vi "BELKIN Read Dest FIFO.vi"(7 "Read Timeout (ms)":i32=5000, 8 "error in (no error)":errorcluster, 9 "FPGA VI Reference In":refnum<k20>, 10 "Maximum Pixels per Read":i32=-1, 11 "Image":T1) -> (0 "error out":errorcluster, 1 "FPGA VI Reference Out":refnum<k20>, 3 "Image Out":T1)   [LabVIEW 2015]
doc: "Transfers an image from the target FPGA to the host processor via DMA FIFO."
uses:
  <vilib>/vision/Image Controls.llb/IMAQ Image.ctl
  <vilib>/rvi/errors/niLvFpgaAdjustHostInterfaceError.vi
  <vilib>/rvi/interface/nirviMethod/nirviMethod.xnode
  <vilib>/rvi/errors/niLvFpgaMergeErrorWithErrorCode.vi
  <vilib>/vision/EDVR.llb/IMAQ ImageToEDVR 2D U8.vi
  nivissvc.dll
  <vilib>/FPGAPlugInAG/Dynamic/niLvFpga_ReadFifo_Dynamic.vi
  <vilib>/FPGAPlugInAG/Dynamic/niLvFpga_AcquireReadRegionFifo_Dynamic.vi
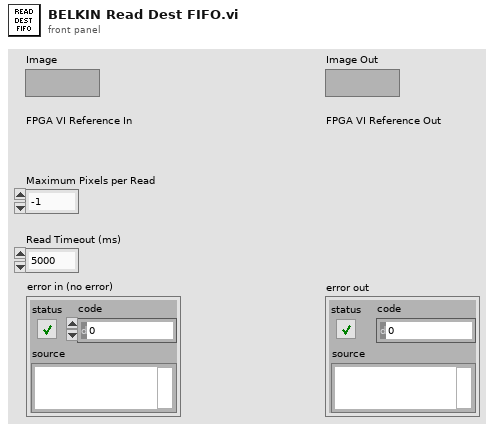
[diagram p1: front panel]
types:
  T1 = typedef "IMAQ Image.ctl" = refnum<image>
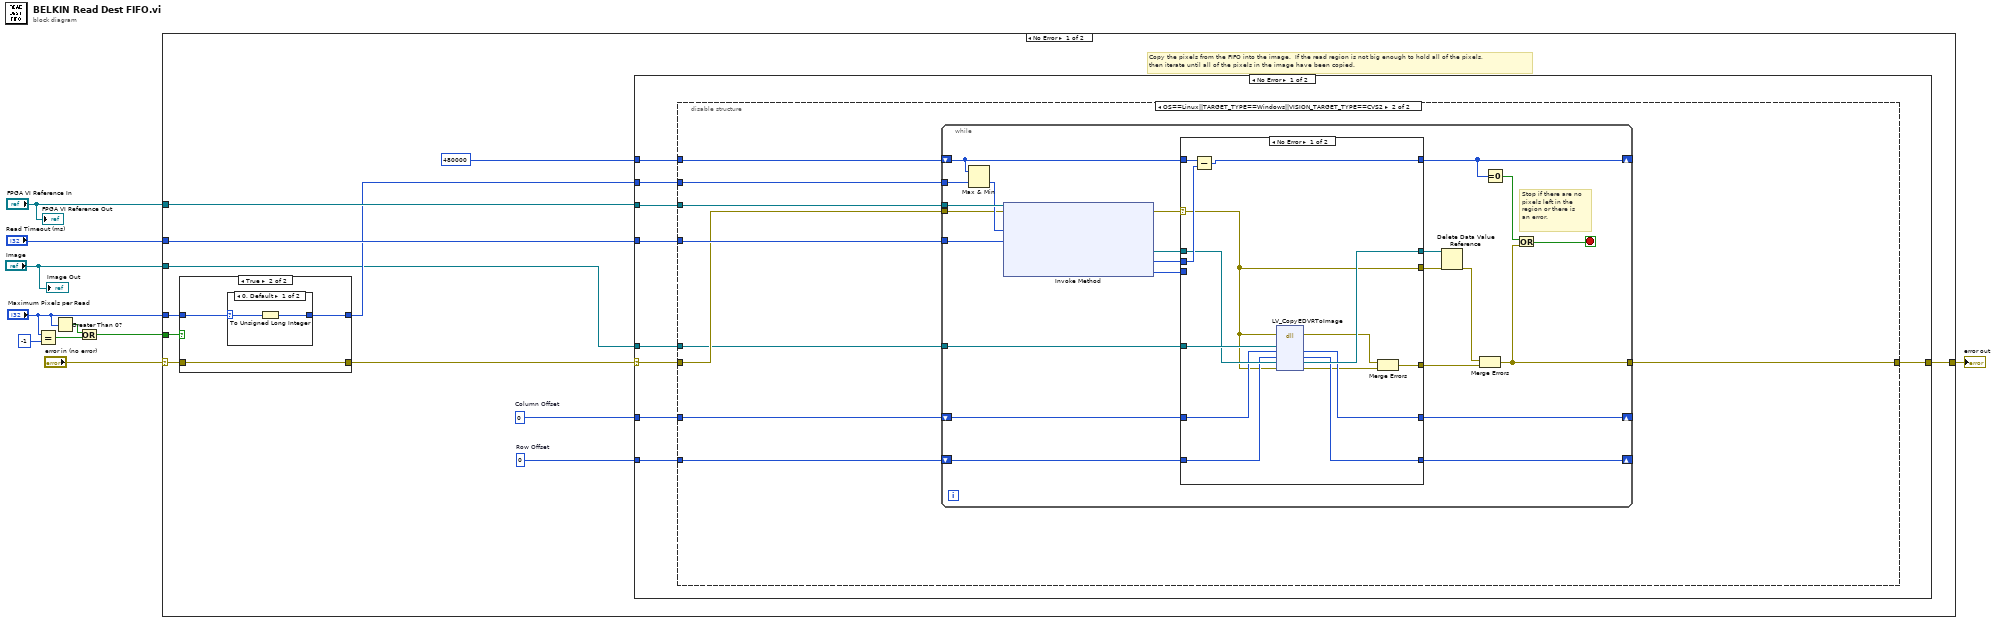
[diagram p0: block diagram]
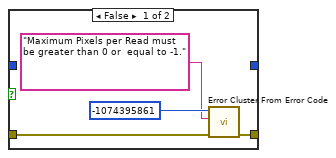
[diagram p2: hidden frame]
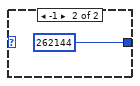
[diagram p3: hidden frame]
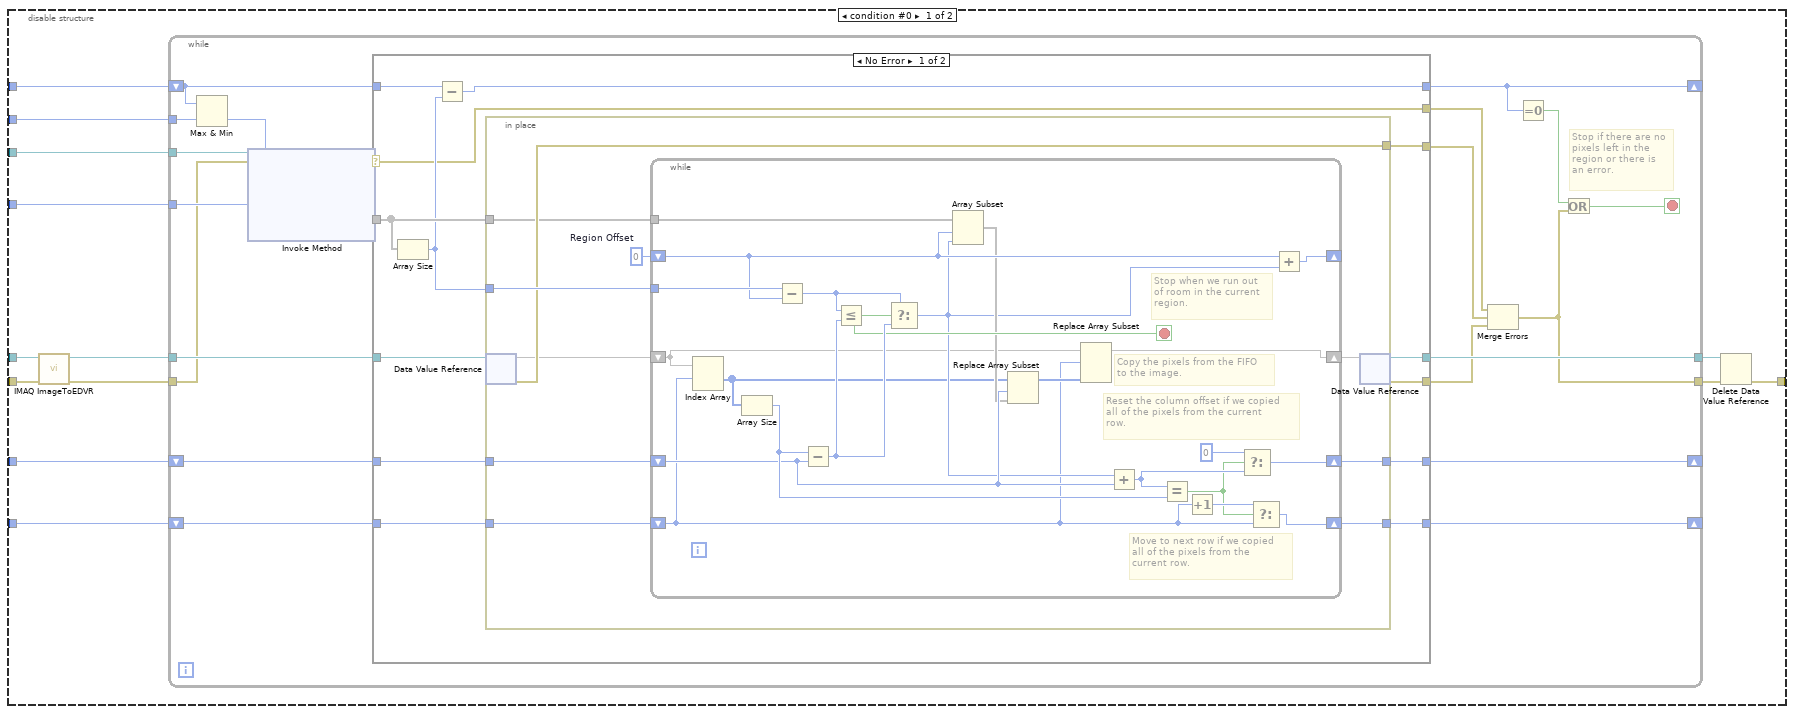
[diagram p4: hidden frame]
diagram:
  n1 = Equal?(x="Maximum Pixels per Read", y=-1) -> (x = y?=w6:bool)
  n2 = Greater Than 0?(x="Maximum Pixels per Read") -> (x > 0?=w7:bool)
  n3 = Or(x=w7, y=w6) -> (x .or. y?=w5:bool)
  n4 = case shown="No Error" "error in (no error)" {
    selector: "error in (no error)" -> [w12 w178]
    tunnel: "FPGA VI Reference In" -> [w20 _]
    tunnel: "Read Timeout (ms)" -> [w19 _]
    tunnel: w5 -> [w18 _]
    tunnel: "Maximum Pixels per Read" -> [w17 _]
    tunnel: "Image" -> [w14 _]
    tunnel: [w13 w178] -> w2
    frame No Error {
      w21 = u32 0  # Row Offset
      w22 = u32 0  # Column Offset
      # "Copy the pixels from the FIFO into the image.  If the read region is not big enough to hold all of the pixels,\nthen iterate until all of the pixels in the image have been copied."
      n5 = case shown="True" w18 {
        tunnel: w12 -> [w24 w29]
        tunnel: [w23 w29] -> w16
        tunnel: w17 -> [_ w28]
        tunnel: [_ w27] -> w15
        frame False {
          n6 = call <vilib>:"Error Cluster From Error Code.vi"("error in (no error)"=w24, "error message (\"\")"="Maximum Pixels per Read must be greater than 0 or  equal to -1." ("error message (\"\")"), "error code (0)"=-1074395861) -> ("error out"=w23:errorcluster)  [unwired: 6 in]
        }
        frame True {
          n7 = case shown="0, Default" w28 {
            selector: w28 -> [w31 _]
            tunnel: [w30 u32 262144 ("Maximum Pixels per Write")] -> w27
            frame 0, Default {
              n8 = To Unsigned Long Integer(number=w31) -> (unsigned 32bit integer=w30:u32)
            }
            frame -1 {
            }
          }
        }
      }
      n9 = case shown="No Error" w16 {
        selector: w16 -> [w40 w177]
        tunnel: 480000 ("x*y") -> [w34 _]
        tunnel: w22 -> [w39 _]
        tunnel: w21 -> [w38 _]
        tunnel: w20 -> [w36 _]
        tunnel: [w33 w177] -> w13
        tunnel: w15 -> [w35 _]
        tunnel: w19 -> [w37 _]
        tunnel: w14 -> [w41 _]
        frame No Error {
          n10 = disable-structure shown="OS==Linux||TARGET_TYPE==Windows||VISION_TARGET_TYPE==CVS2" {
            disable-tunnel: w34 -> [w54 w134]
            disable-tunnel: w39 -> [w53 w133]
            disable-tunnel: w38 -> [w52 w132]
            disable-tunnel: w36 -> [w51 w131]
            disable-tunnel: [w42 w130] -> w33
            disable-tunnel: w35 -> [w50 w129]
            disable-tunnel: w37 -> [w49 w128]
            disable-tunnel: w41 -> [w48 w126]
            disable-tunnel: w40 -> [w46 w127]
            frame condition #0 {
              n11 = call-poly <vilib>:"IMAQ ImageToEDVR.vi"("error in (no error)"=w46, "Image"=w48) -> ("error out"=w45:errorcluster, "EDVR 2D U8"=w47:refnum<data-value>)  [unwired: 7 in, 1 out]
              n12 = while {
                shift-right: [w66] -> _
                shift-left: w54 -> [w62]
                shift-right: [w71] -> _
                shift-left: w53 -> [w73]
                shift-right: [w74] -> _
                shift-left: w52 -> [w72]
                tunnel: w51 -> [w70]
                tunnel: [w68] -> w44
                tunnel: [w64] -> w43
                tunnel: w50 -> [w60]
                tunnel: w49 -> [w59]
                tunnel: w47 -> [w56]
                tunnel: w45 -> [w55]
                stop <- w65 stop-if-true
                # "Stop if there are no\npixels left in the \nregion or there is\nan error."
                n13 = Max & Min(x=w62, y=w60) -> (min(x,y)=w61:u32)  [unwired: 1 out]
                n14 = xnode "Invoke Method"("FPGA VI Reference In"=w70, "error in"=w55, "Number of Elements"=w61, "Timeout (ms)"=w59) -> ("error out"=w69:errorcluster, "Data"=w75:void[])  [unwired: 2 out]
                n15 = case shown="No Error" w69 {
                  selector: w69 -> [w76 w121]
                  tunnel: w62 -> [w88 w124]
                  tunnel: [w87 w124] -> w66
                  tunnel: w56 -> [w86 w125]
                  tunnel: w75 -> [w78 _]
                  tunnel: [w85 w122] -> w74
                  tunnel: w73 -> [w84 w123]
                  tunnel: w72 -> [w83 w122]
                  tunnel: [w82 w123] -> w71
                  tunnel: [w81 w125] -> w68
                  tunnel: [w76 w121] -> w58
                  tunnel: [w80 _] -> w57
                  tunnel: [w79 _] -> w67
                  frame No Error {
                    n16 = Array Size(array=w78) -> (size(s)=w77:i32)
                    n17 = Subtract(x=w88, y=w77) -> (x-y=w87:i32)
                    n18 = in-place {
                      in-place-border: w77 -> [w96]
                      in-place-border: [w98] -> w85
                      in-place-border: w84 -> [w95]
                      in-place-border: w83 -> [w91]
                      in-place-border: [w94] -> w82
                      in-place-border: [w93] -> w79
                      in-place-border: w78 -> [w89]
                      w97 = u32 0  # Region Offset
                      n19 = in-place-dvr #1(w86) -> (w92:u8[][], w93:errorcluster)
                      n20 = while {
                        shift-right: [w118] -> _
                        shift-left: w97 -> [w117]
                        tunnel: w89 -> [w107]
                        tunnel: w96 -> [w120]
                        shift-right: [w112] -> w94
                        shift-left: w95 -> [w108]
                        shift-right: [w99] -> w90
                        shift-left: w92 -> [w102]
                        shift-right: [w110] -> w98
                        shift-left: w91 -> [w100]
                        stop <- w109 stop-if-true
                        # "Stop when we run out\nof room in the current\nregion."
                        # "Copy the pixels from the FIFO\nto the image."
                        # "Reset the column offset if we copied\nall of the pixels from the current\nrow."
                        # "Move to next row if we copied\nall of the pixels from the\ncurrent row."
                        n21 = Index Array(array=w102, index (row)=w100) -> (element=w103:u8[])  [unwired: 1 in]
                        n22 = Array Size(array=w103) -> (size(s)=w116:i32)
                        n23 = Subtract(x=w120, y=w117) -> (x-y=w119:u32)
                        n24 = Subtract(x=w116, y=w108) -> (x-y=w115:u32)
                        n25 = Less Or Equal?(x=w119, y=w115) -> (x <= y?=w109:bool)
                        n26 = Select(t=w119, s=w109, f=w115) -> (s? t:f=w105:u32)
                        n27 = Array Subset(array=w107, index=w117, length=w105) -> (w106:void[])
                        n28 = Replace Array Subset(array=w103, new element=w106, index=w108) -> (w101:u8[])
                        n29 = Replace Array Subset(array=w102, new element=w101, index (row)=w100) -> (w99:u8[][])  [unwired: 1 in]
                        n30 = Add(x=w105, y=w108) -> (x+y=w113:u32)
                        n31 = Equal?(x=w113, y=w116) -> (x = y?=w104:bool)
                        n32 = Increment(x=w100) -> (x+1=w111:u32)
                        n33 = Select(t=u32 0 ("Elements In Region"), s=w104, f=w113) -> (s? t:f=w112:u32)
                        n34 = Select(t=w111, s=w104, f=w100) -> (s? t:f=w110:u32)
                        n35 = Add(x=w117, y=w105) -> (x+y=w118:u32)
                      }
                      n36 = in-place-dvr #1(w90) -> (w81:refnum<data-value>, w80:errorcluster)
                    }
                  }
                  frame Error {
                  }
                }
                n37 = Merge Errors(w58, w67, w57) -> (w64:errorcluster)
                n38 = Equal To 0?(x=w66) -> (x = 0?=w63:bool)
                n39 = Or(x=w63, y=w64) -> (x .or. y?=w65:bool)
              }
              n40 = Delete Data Value Reference(data value reference=w44, error in=w43) -> (error out=w42:errorcluster)  [unwired: 1 out]
            }
            frame condition #1 (active) {
              n41 = while {
                shift-right: [w148] -> _
                shift-left: w134 -> [w145]
                shift-right: [w152] -> _
                shift-left: w133 -> [w154]
                shift-right: [w155] -> _
                shift-left: w132 -> [w153]
                tunnel: w131 -> [w151]
                tunnel: [w135] -> w130
                tunnel: w129 -> [w142]
                tunnel: w128 -> [w141]
                tunnel: w127 -> [w140]
                tunnel: w126 -> [w139]
                stop <- w147 stop-if-true
                # "Stop if there are no\npixels left in the \nregion or there is\nan error."
                n42 = Max & Min(x=w145, y=w142) -> (min(x,y)=w144:u32)  [unwired: 1 out]
                n43 = xnode "Invoke Method"("FPGA VI Reference In"=w151, "error in"=w140, "Number of Elements"=w144, "Timeout (ms)"=w141) -> ("error out"=w150:errorcluster, "Read Region Reference"=w157:refnum<data-value>, "Elements In Region"=w156:u32, "Elements Remaining"=w143:u32)  [unwired: 1 out]
                n44 = case shown="No Error" w150 {
                  selector: w150 -> [w158 w172]
                  tunnel: w145 -> [w171 w176]
                  tunnel: [w170 w176] -> w148
                  tunnel: w157 -> [w166 w173]
                  tunnel: w156 -> [w167 _]
                  tunnel: [w162 w174] -> w155
                  tunnel: w154 -> [w165 w175]
                  tunnel: w153 -> [w164 w174]
                  tunnel: [w163 w175] -> w152
                  tunnel: [w168 w173] -> w149
                  tunnel: [w158 w172] -> w138
                  tunnel: w143 -> [_ _]
                  tunnel: w139 -> [w169 _]
                  tunnel: [w159 w172] -> w137
                  frame No Error {
                    n45 = Subtract(x=w171, y=w167) -> (x-y=w170:u32)
                    n46 = dll-call lib="nivissvc.*" fn="LV_CopyEDVRToImage"(error in=w158, "image"=w169, "xImageOffset"=w165, "yImageOffset"=w164, "EDVR"=w166, "error"=w158) -> (error out=w160:errorcluster, "xImageOffset"=w163:u32, "yImageOffset"=w162:u32, "EDVR"=w168:refnum<data-value>, "error"=w161:errorcluster)  [unwired: 4 in, 1 out]
                    n47 = Merge Errors(w160, w161) -> (w159:errorcluster)
                  }
                  frame Error {
                  }
                }
                n48 = Delete Data Value Reference(data value reference=w149, error in=w138) -> (error out=w136:errorcluster)  [unwired: 1 out]
                n49 = Merge Errors(w136, w137) -> (w135:errorcluster)
                n50 = Equal To 0?(x=w148) -> (x = 0?=w146:bool)
                n51 = Or(x=w146, y=w135) -> (x .or. y?=w147:bool)
              }
            }
          }
        }
        frame Error {
        }
      }
    }
    frame Error {
    }
  }
  "error out" <- w2
  "Image Out" <- "Image"
  "FPGA VI Reference Out" <- "FPGA VI Reference In"
